vi "Index Rune.vi"(8 "error in (no error)":errorcluster, 10 "Byte Offset":i32, 11 "UTF8 in":refnum<class "UTF-8 String.lvclass">) -> (0 "error out":errorcluster, 2 "Rune":u32, 3 "UTF8 out":refnum<class "UTF-8 String.lvclass">)   [LabVIEW 2019, in "JKI Unicode.lvlib" / "UTF-8 String.lvclass"]
doc: "JKI Unicode 1.0.0.7\nTomi Maila - JKI\nCopyright (c) 2016, JKI"
uses:
  UTF-8 String.lvclass
  UTF-8 String.lvclass/UTF-8 String.ctl
  Bytes In Rune.vi
  <vilib>/Utility/error.llb/Error Cluster From Error Code.vi
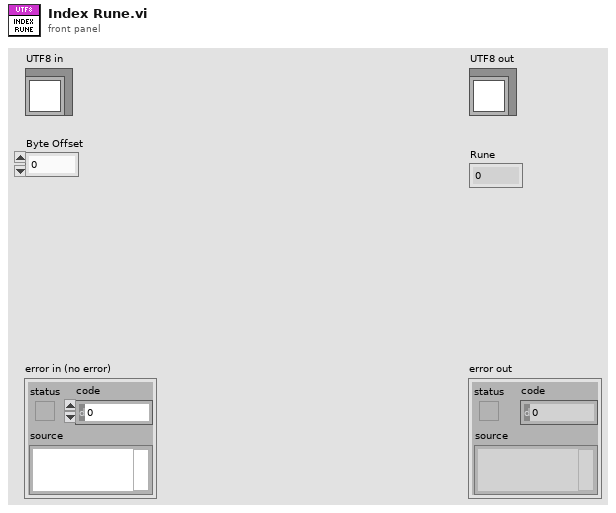
[diagram p1: front panel]
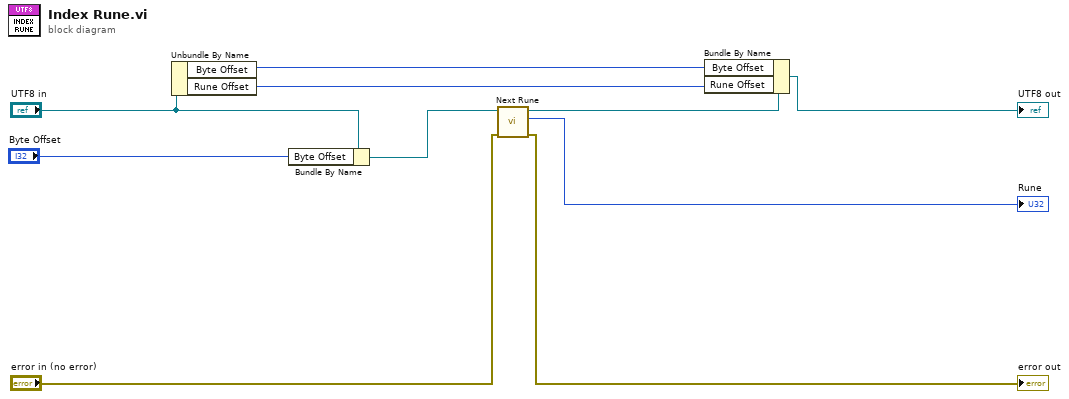
[diagram p0: block diagram]
diagram:
  n1 = Unbundle By Name("UTF8 in") -> ("Byte Offset"=w5:i32, "Rune Offset"=w4:i32)
  n2 = Bundle By Name(cluster="UTF8 in", "Byte Offset"="Byte Offset") -> (w2:refnum<class "UTF-8 String.lvclass">)
  n3 = call "Next Rune.vi"("error in (no error)"="error in (no error)", "UTF8 in"=w2) -> ("error out"=→"error out":errorcluster, "Rune"=→"Rune":u32, "UTF8 out"=w7:refnum<class "UTF-8 String.lvclass">)  [unwired: 7 in]
  n4 = Bundle By Name(cluster=w7, "Byte Offset"=w5, "Rune Offset"=w4) -> (→"UTF8 out":refnum<class "UTF-8 String.lvclass">)
